vi "Actor Core.vi"(8 "error in":errorcluster, 11 "OneButtonDialogBox In":refnum<class "OneButtonDialogBox.lvclass">) -> (0 "error out":errorcluster, 3 "Actor out":refnum<class "Actor.lvclass">)   [LabVIEW 2015, in "OneButtonDialogBox.lvlib" / "OneButtonDialogBox.lvclass"]
doc: "(<B>Filename</B>: Actor Framework.lvlib:Actor.lvclass:Actor Core.vi)\n\nReceives messages to the actor, reacts to them, and initiates any error handling that may shut the actor down.\n\nDescendant classes may override this VI to append parallel tasks for the actor to complete while it handles messages. Overrides use the Call Parent Method node."
uses:
  OneButtonDialogBox.lvclass
  <vilib>/ActorFramework/Actor/Actor.lvclass
  <vilib>/ActorFramework/Actor/Actor.lvclass/Actor.ctl
  <vilib>/ActorFramework/Message Enqueuer/Message Enqueuer.lvclass/Message Enqueuer.ctl
  OneButtonDialogBox.lvclass/OneButtonDialogBox.ctl
  <vilib>/ActorFramework/Message Enqueuer/Init from Existing Queue.vi
  IDialogBox/IDialogBox/IDialogBox.lvclass
  <vilib>/ActorFramework/Message Enqueuer/Message Enqueuer.lvclass
  AutoRegistration/ActorAutoRegistration/ActorAutoRegistration.lvclass
panel:
  out "Message Text":string
  in  "Okay":bool
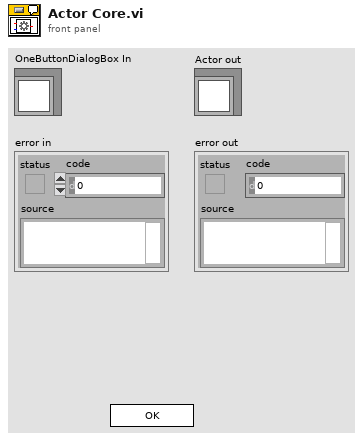
[diagram p1: front panel]
types:
  T1 = enum32{"Invalid", "Default", "Floating", "Floating/Auto-Hide", "Modal"}
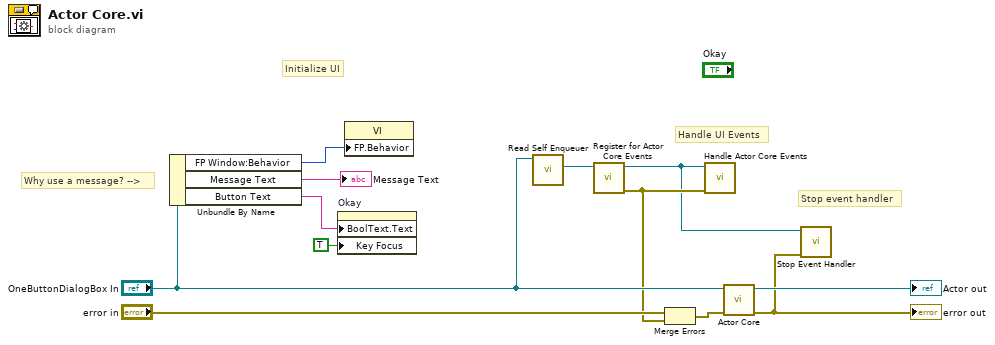
[diagram p0: block diagram]
diagram:
  # "Initialize UI"
  # "Stop event handler"
  # "Handle UI Events"
  # "Why use a message? -->"
  n1 = Unbundle By Name("OneButtonDialogBox In") -> ("FP Window:Behavior"=w8:T1, "Message Text"=→"Message Text":string, "Button Text"=w10:string)
  n2 = property on="Okay" class="Bool"("BoolText.Text"=w10, "Key Focus"=TRUE) -> ()  [unwired: 2 in, 2 out]
  n3 = property class="VI"("FP.Behavior"=w8) -> ()  [unwired: 2 in, 2 out]
  n4 = call <vilib>:"Read Self Enqueuer.vi"("Actor"="OneButtonDialogBox In") -> ("Self Enqueuer"=w7:refnum<class "Message Enqueuer.lvclass">)  [unwired: 10 in]
  n5 = call "Register for Actor Core Events.vi"("Actor Enqueuer"=w7) -> ("error out"=w2:errorcluster, "ActorAutoRegistration Out"=w1:refnum<class "ActorAutoRegistration.lvclass">)  [unwired: 9 in]
  n6 = Merge Errors("error in", w2) -> (w5:errorcluster)
  n7 = call-dynamic "Handle Actor Core Events.vi"("error in (no error)"=w2, "ActorAutoRegistration in"=w1) -> ()  [unwired: 9 in, 1 out]
  n8 = call-parent "Actor Core.vi"("error in"=w5, "IViewable In"="OneButtonDialogBox In") -> ("error out"=w3:errorcluster, "Actor out"=→"Actor out":refnum<class "Actor.lvclass">)  [unwired: 8 in]
  "error out" <- w3
  n9 = call-dynamic "Stop Event Handler.vi"("error in (no error)"=w3, "ActorAutoRegistration in"=w1) -> ()  [unwired: 9 in, 1 out]
